vi "开机连接.vi"(8 "error in":errorcluster, 10 "波特率":u32=19200, 11 "串口号":refnum<visa-resource-name>) -> (0 "error out":errorcluster, 1 "连接成功":bool, 3 "serial master instance":refnum<class "Modbus Master.lvclass">)   [LabVIEW 2020]
uses:
  <vilib>/NI/Modbus Library/API/Master/Modbus Master.lvclass
  <vilib>/NI/Modbus Library/API/Wrapper/Create Serial Master.vi
  <vilib>/NI/Modbus Library/API/Wrapper/API Main.lvlib
panel:
  out "文本提示":string
  in  "ID站号":u8=1
  in  "校验位":u16(ring) items=["None", "Odd", "Even", "Mark", "Space"]
  in  "传输模式":enum16{"RTU", "ASCII"}(ring)
  in  "流控制":u16(ring) items=["None", "XON/XOFF", "RTS/CTS", "XON/XOFF & RTS/CTS", "DTR/DSR", "XON/XOFF & DTR/DSR"]
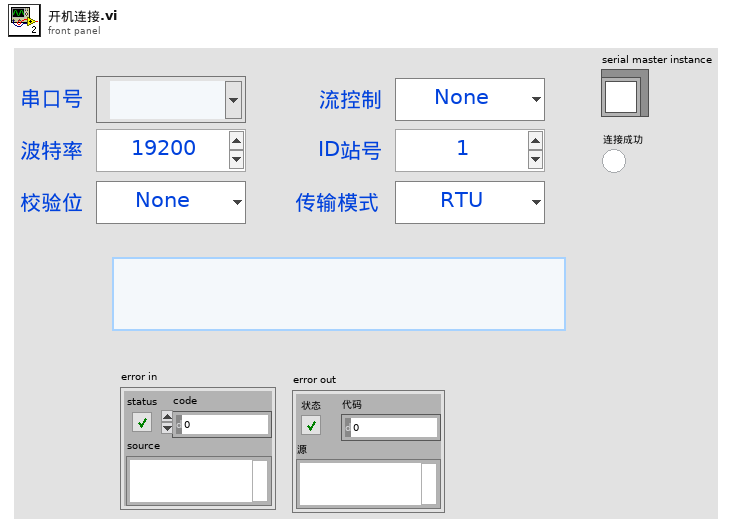
[diagram p1: front panel]
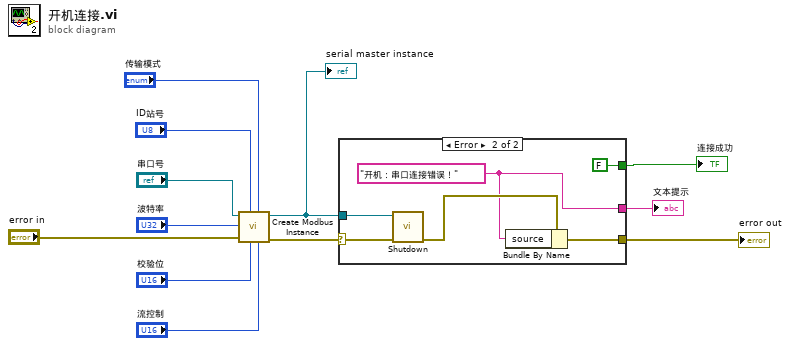
[diagram p0: block diagram]
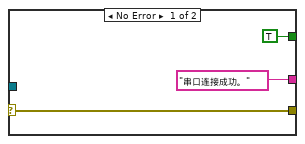
[diagram p2: hidden frame]
diagram:
  n1 = call-poly <vilib>:"Create Modbus Instance.vi"("flow control (none)"="流控制", "serial type"="传输模式", "parity (even)"="校验位", "unit ID"="ID站号", "error in"="error in", "baud rate"="波特率", "VISA resource name"="串口号") -> ("error out"=w7:errorcluster, "serial master instance"=w6:refnum<class "Modbus Master.lvclass">)  [unwired: 3 in]
  "serial master instance" <- w6
  n2 = case shown="Error" w7 {
    selector: w7 -> [w15 w20]
    tunnel: w6 -> [_ w19]
    tunnel: [w15 w16] -> w1
    tunnel: ["串口连接成功。" ("消息") w17] -> w4
    tunnel: [TRUE FALSE] -> w5
    frame No Error {
    }
    frame Error {
      w17 = "开机：串口连接错误！" ("消息")
      n3 = call-dynamic "Shutdown.vi"("error in"=w20, "Modbus master in"=w19) -> ("error out"=w18:errorcluster)  [unwired: 9 in]
      n4 = Bundle By Name(cluster=w18, "source"=w17) -> (w16:errorcluster)
    }
  }
  "连接成功" <- w5
  "文本提示" <- w4
  "error out" <- w1
